vi "Call_Video_Still_with_Averaging.vi"() -> (0 "Error out":errorcluster)   [LabVIEW 2015]
uses:
  Anemometry Sub Vis/Globals/Trav_pos_global.vi
  Anemometry Sub Vis/Globals/Meas_global.vi
  Camera Server/Globals/CamServer global.vi
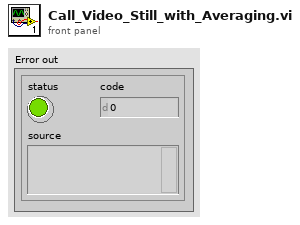
[diagram p1: front panel]
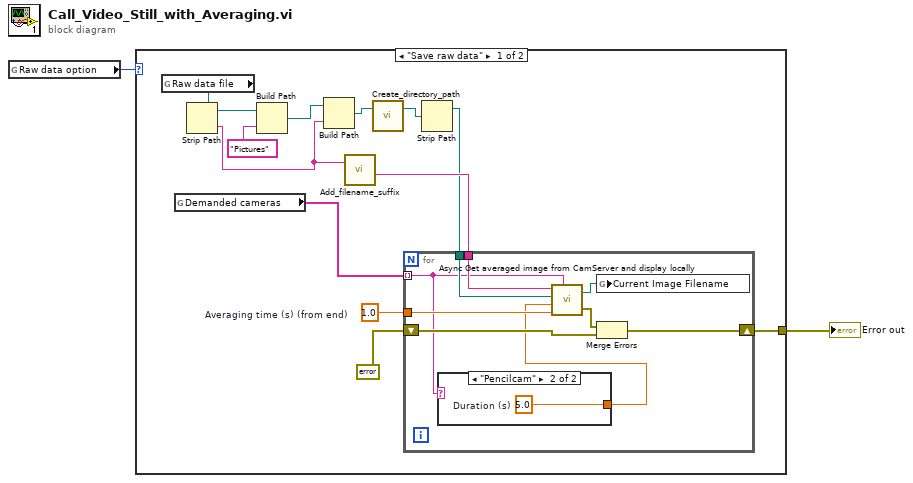
[diagram p0: block diagram]
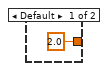
[diagram p2: hidden frame]
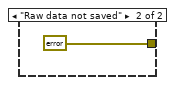
[diagram p3: hidden frame]
diagram:
  n1 = global read "Meas_global.vi" "Raw data option"() -> (w2:enum16{"Save raw data", "Raw data not saved"})
  n2 = case shown="\"Save raw data\"" w2 {
    tunnel: [w3 errorcluster {"status"=FALSE, "code"=0, "source"=""} ("Error out")] -> w1
    frame "Save raw data" {
      w6 = 1.0  # Averaging time (s) (from end)
      n3 = global read "Meas_global.vi" "Raw data file"() -> (w13:path)
      n4 = global read "CamServer global.vi" "Demanded cameras"() -> (w4:string[])
      n5 = Strip Path(path=w13) -> (stripped path=w15:path, name=w9:string)
      n6 = Build Path(base path=w15, name or relative path="Pictures") -> (appended path=w12:path)
      n7 = Build Path(base path=w12, name or relative path=w9) -> (appended path=w11:path)
      n8 = call "Add_filename_suffix.vi"("Filename"=w9) -> ("Base name"=w8:string)  [unwired: 1 in, 3 out]
      n9 = call "Create_directory_path.vi"("Path name"=w11) -> ("Path name Out"=w10:path)  [unwired: 1 in, 1 out]
      n10 = Strip Path(path=w10) -> (stripped path=w7:path)  [unwired: 1 out]
      n11 = for {
        tunnel: w8 -> [w23]
        tunnel: w7 -> [w22]
        tunnel: w6 -> [w21]
        shift-right: [w18] -> w3
        shift-left: errorcluster {"status"=FALSE, "code"=0, "source"=""} ("Error out") -> [w20]
        tunnel: w4 -> [w17] mode=indexing
        n12 = case shown="\"Pencilcam\"" w17 {
          tunnel: [2.0 ("Duration (s)") w26] -> w16
          frame Default {
          }
          frame "Pencilcam" {
            w26 = 5.0  # Duration (s)
          }
        }
        n13 = call "Async Get averaged image from CamServer and display locally.vi"("Camera"=w17, "Averaging time (s) (from end)"=w21, "Duration (s)"=w16, "Image directory path"=w22, "Image name"=w23) -> ("Error out"=w19:errorcluster, "Image file path"=w24:path)  [unwired: 1 in]
        n14 = global write "Trav_pos_global.vi" "Current Image Filename"(w24) -> ()
        n15 = Merge Errors(w19, w20) -> (w18:errorcluster)
      }
    }
    frame "Raw data not saved" {
    }
  }
  "Error out" <- w1
